vi "FGV Dichtheitstest.vi"(6 "Aktionen":T1, 8 "Dichtheitstest?":u16, 10 "Aktionen Dichtheitstest":T2) -> (0 "Dichtheitstest?":bool, 2 "Aktionen Dichtheitstest":T2)   [LabVIEW 2020, in "Allgemein.lvlib"]
uses:
  Allgemein.lvlib
  Seiten/Erweiterte Konfig/Aktionen Dichtheitstest.ctl
  Aktionen FGV Dichtheitstest.ctl
  Seiten/Erweiterte Konfig/Erweiterte Konfig.lvlib
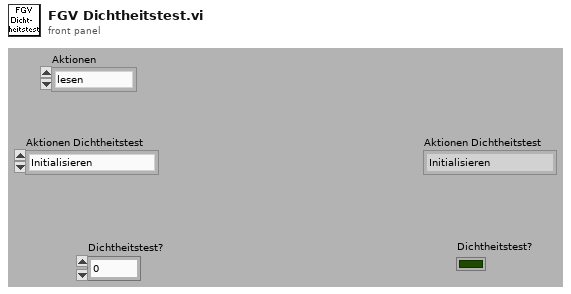
[diagram p1: front panel]
types:
  T1 = typedef "Allgemein.lvlib/Aktionen FGV Dichtheitstest.ctl" = enum16{"lesen", "schreiben"}
  T2 = typedef "Erweiterte Konfig.lvlib/Aktionen Dichtheitstest.ctl" = enum16{"Initialisieren", "Unterdruck aufbauen", "Prop schließen", "Warten", "Auswertung", "Fertig"}
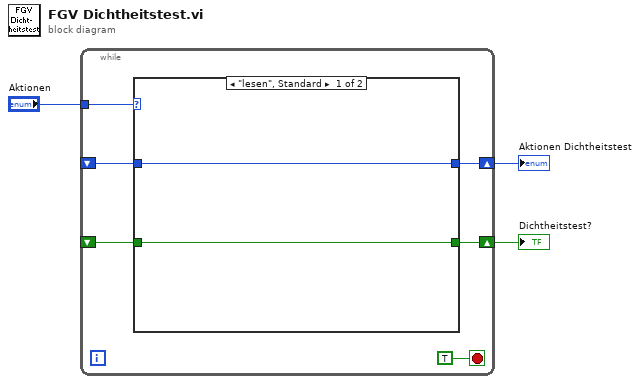
[diagram p0: block diagram]
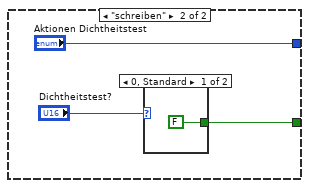
[diagram p2: hidden frame]
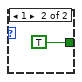
[diagram p3: hidden frame]
diagram:
  n1 = while {
    tunnel: "Aktionen" -> [w8]
    shift-right: [w7] -> w1
    shift-left: _ -> [w5]
    shift-right: [w6] -> w2
    shift-left: _ -> [w4]
    stop <- TRUE stop-if-true
    n2 = case shown="\"lesen\", Standard" w8 {
      tunnel: [w11 "Aktionen Dichtheitstest"] -> w7
      tunnel: [w10 w12] -> w6
      tunnel: w5 -> [w11 _]
      tunnel: w4 -> [w10 _]
      frame "lesen", Default {
      }
      frame "schreiben" {
        n3 = case shown="0, Standard" "Dichtheitstest?" {
          tunnel: [FALSE TRUE] -> w12
          frame 0, Default {
          }
          frame 1 {
          }
        }
      }
    }
  }
  "Aktionen Dichtheitstest" <- w1
  "Dichtheitstest?" <- w2
